vi "Disconnect.vi"(8 "error in":errorcluster, 11 "IgusMotorDrive in":refnum<class "IgusMotorDrive.lvclass">) -> (0 "error out":errorcluster, 3 "IgusMotorDrive out":refnum<class "IgusMotorDrive.lvclass">)   [LabVIEW 2016, in "IgusMotorDrive.lvclass"]
uses:
  IgusMotorDrive.lvclass
  C:/Projekte/Lufft/CHM8K/igus Stages/igusPositioningSystem/Modules/Classes/motor-drive/MotorDrive.lvclass
  IgusMotorDrive.lvclass/IgusMotorDrive.ctl
  Libraries/Modbus-Master/MB_Master_TCP/MB_Master_TCP.lvclass
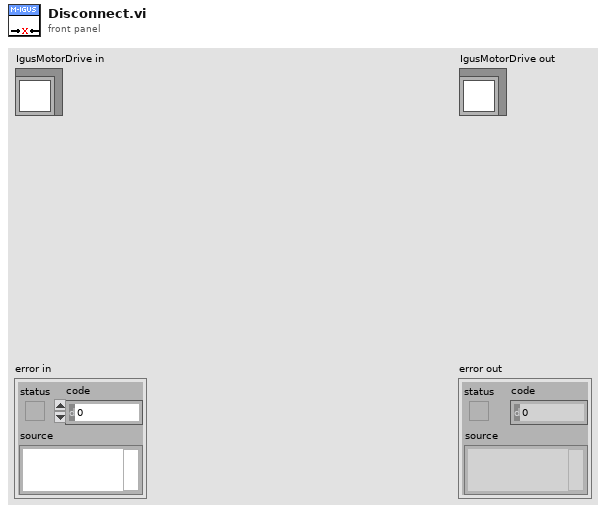
[diagram p1: front panel]
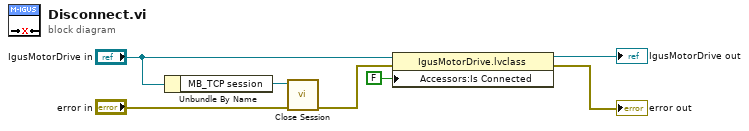
[diagram p0: block diagram]
diagram:
  n1 = Unbundle By Name("IgusMotorDrive in") -> ("MB_TCP session"=w6:refnum<class "MB_Master_TCP.lvclass">)
  n2 = call-dynamic "Close Session.vi"("error in (no error)"="error in", "MB TCP session"=w6) -> ("error out"=w5:errorcluster)  [unwired: 9 in]
  n3 = property class="IgusMotorDrive.lvclass"(reference="IgusMotorDrive in", error in=w5, "Accessors:Is Connected"=FALSE ("Is Connected")) -> (reference out=→"IgusMotorDrive out":refnum<class "IgusMotorDrive.lvclass">, error out=→"error out":errorcluster)
